vi "Upload File to Bucket.vi"() -> ()   [LabVIEW 2015]
doc: "Demonstrates how to upload a file from the local file system to an Amazon S3 bucket."
uses:
  <vilib>/AWS Toolkit/Core/HTTP Request/AWS Credentials.ctl
  <vilib>/AWS Toolkit/S3/ACL.ctl
  <vilib>/AWS Toolkit/S3/PUT Object Request Parameters.ctl
  <vilib>/AWS Toolkit/S3/Storage Class.ctl
  <vilib>/AWS Toolkit/Core/HTTP Request/Name Value Pair.ctl
  <vilib>/AWS Toolkit/Core/HTTP Request/HTTP Request.lvclass
  <vilib>/AWS Toolkit/S3/Bucket/Bucket.lvclass
  <vilib>/AWS Toolkit/S3/NI_AWS_S3.lvlib
panel:
  in  "File to Upload":path
  in  "Secret Key":string
  in  "Access Key":string
  out "New Object Location":string
  in  "Public":bool
  in  "Object Path":string="uploads/"
  in  "Destination Bucket":string
  # "Overview: Demonstrates how to upload a file to an Amazon S3 bucket.\nRequirements: NI Cloud Toolkit for AWS and a registered Amazon AWS account\nInstructions:\n1. Specify the Access Key and Secret Key for your AWS account. You can create an account at http://aws.amazon.com.\n2. Specify a Destination Bucket for the file. If you have not created a bucket, you can run the Create New Bucket.vi example to create a new bucket.\n3. Set Public to TRUE if you want the file to be public.\n4. Specify the File to Upload.\n5. Set the Object Path if you want to store the file in a folder within the bucket.\n6. Run the VI. Observe the URL of the stored file in the New Object Location indicator."
  # "Note: If you set Public to FALSE, you will not be able to download the file using the New Object Location URL. This is because you must use an authentication method to access non-public objects."
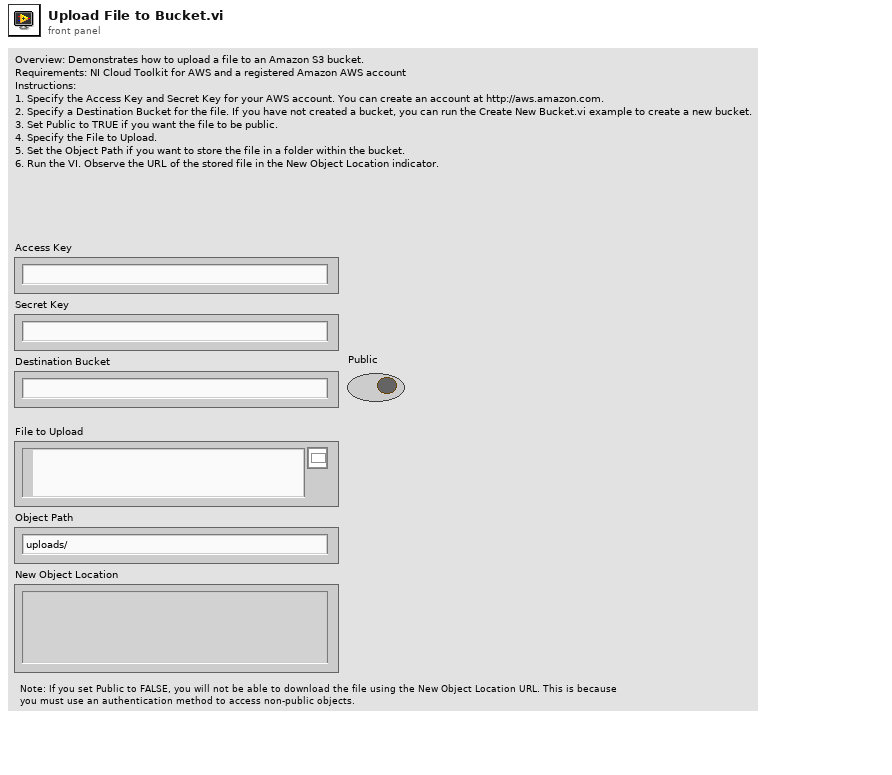
[diagram p1: front panel]
types:
  T1 = typedef "NI_AWS_Core.lvlib/HTTP Request.lvclass/AWS Credentials.ctl" = cluster{"Access Key":string, "Secret Key":string}
  T2 = typedef "NI_AWS_S3.lvlib/ACL.ctl" = enum16{"private", "public-read", "public-read-write", "aws-exec-read", "authenticated-read", "bucket-owner-read", "bucket-owner-full-control"}
  T3 = typedef "NI_AWS_S3.lvlib/PUT Object Request Parameters.ctl" = cluster{"Content Type":string, "ACL":T2, "Storage Class":T4, "User-Defined Metadata":T5[]}
  T4 = typedef "NI_AWS_S3.lvlib/Storage Class.ctl" = enum16{"STANDARD", "REDUCED_REDUNDANCY"}
  T5 = typedef "NI_AWS_Core.lvlib/HTTP Request.lvclass/Name Value Pair.ctl" = cluster{"name":string, "value":string}
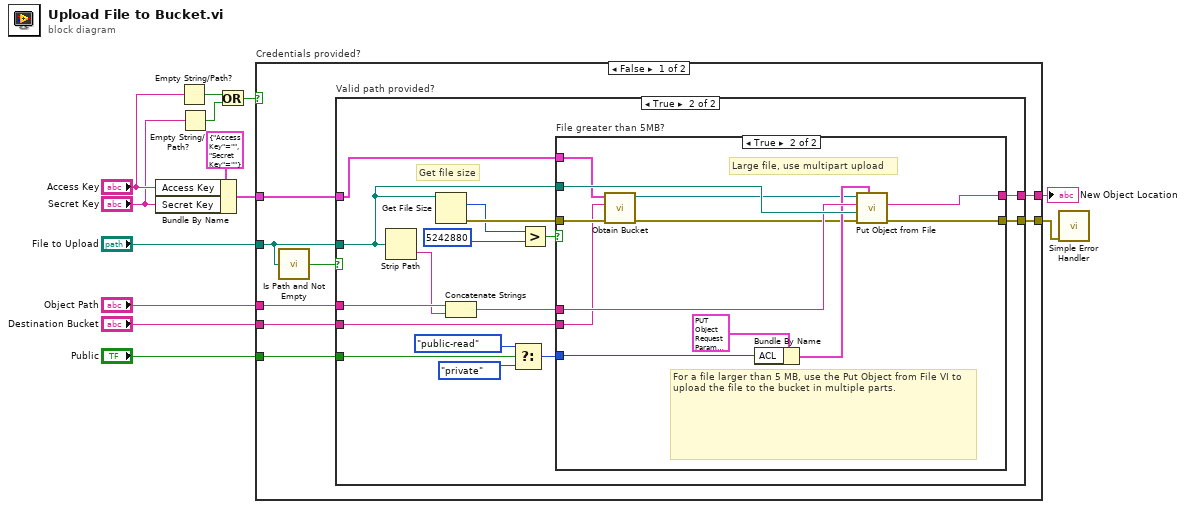
[diagram p0: block diagram]
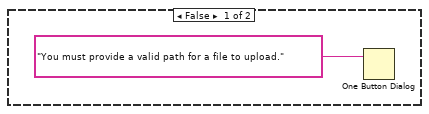
[diagram p2: hidden frame]
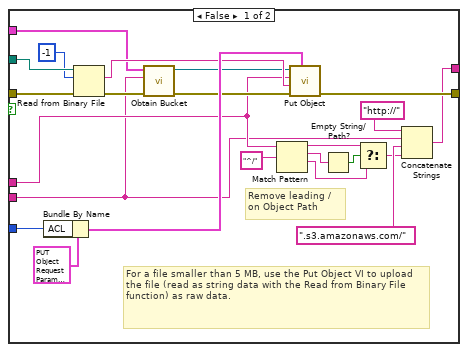
[diagram p3: hidden frame]
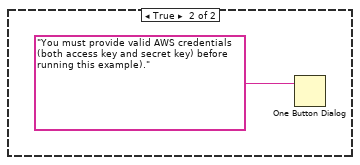
[diagram p4: hidden frame]
diagram:
  n1 = Bundle By Name(cluster=T1 {"Access Key"="", "Secret Key"=""} ("AWS Credentials in"), "Access Key"="Access Key", "Secret Key"="Secret Key") -> (w6:T1)
  n2 = Empty String/Path?(string/path="Access Key") -> (empty?=w11:bool)
  n3 = Empty String/Path?(string/path="Secret Key") -> (empty?=w12:bool)
  n4 = Or(x=w11, y=w12) -> (x .or. y?=w7:bool)
  n5 = case "Credentials provided?" shown="False" w7 {
    tunnel: w6 -> [w20 _]
    tunnel: [w21 _] -> w13
    tunnel: "File to Upload" -> [w19 _]
    tunnel: "Destination Bucket" -> [w17 _]
    tunnel: "Public" -> [w16 _]
    tunnel: "Object Path" -> [w15 _]
    tunnel: [w14 _] -> w1
    frame False {
      n6 = call <vilib>:"Is Path and Not Empty.vi"("path"=w19) -> ("Is Path and Not Empty?"=w18:bool)  [unwired: 4 in]
      n7 = case "Valid path provided?" shown="True" w18 {
        tunnel: w20 -> [_ w23]
        tunnel: w19 -> [_ w27]
        tunnel: [_ w38] -> w21
        tunnel: w17 -> [_ w32]
        tunnel: w16 -> [_ w31]
        tunnel: w15 -> [_ w30]
        tunnel: [_ w26] -> w14
        frame False {
          n8 = One Button Dialog(message="You must provide a valid path for a file to upload.") -> ()  [unwired: 1 in, 1 out]
        }
        frame True {
          # "Get file size"
          n9 = Strip Path(path=w27) -> (name=w28:string)  [unwired: 1 out]
          n10 = Get File Size(file=w27) -> (size (in bytes)=w36:i64, 0:w37:errorcluster)  [unwired: 1 in, 1 out]
          n11 = Concatenate Strings(w30, w28) -> (w29:string)
          n12 = Select(t=ACL."public-read" ("ACL"), s=w31, f=ACL."private" ("ACL")) -> (s? t:f=w33:T2)
          n13 = Greater?(x=w36, y=i64 5242880) -> (0:w34:bool)
          n14 = case "File greater than 5MB?" shown="True" w34 {
            tunnel: w37 -> [w61 w73]
            tunnel: w27 -> [w60 w72]
            tunnel: w32 -> [w40 w63]
            tunnel: w29 -> [w41 w71]
            tunnel: w33 -> [w58 w69]
            tunnel: [w56 w70] -> w26
            tunnel: [w53 w68] -> w38
            tunnel: w23 -> [w42 w64]
            frame False {
              # "Remove leading / \non Object Path"
              # "For a file smaller than 5 MB, use the Put Object VI to upload the file (read as string data with the Read from Binary File function) as raw data."
              n15 = Bundle By Name(cluster=T3 {"Content Type"="binary/octet-stream", "ACL"=enum."private", "Storage Class"=enum."STANDARD", "User-Defined Metadata"=[]} ("PUT Object Request Parameters"), "ACL"=w58) -> (w57:T3)
              n16 = Read from Binary File(8:w61, 10:-1 ("count (1)"), 11:w60) -> (0:w44:errorcluster, 2:w45:string)  [unwired: 3 in, 2 out]
              n17 = call <vilib>:"Obtain Bucket.vi"("error in (no error)"=w44, "Bucket name"=w40, "AWS Credentials"=w42) -> ("error out"=w43:errorcluster, "Bucket"=w39:refnum<class "Bucket.lvclass">)  [unwired: 7 in]
              n18 = Match Pattern(string=w41, regular expression="^/") -> (before substring=w51:string, match substring=w49:string, after substring=w52:string)  [unwired: 1 in, 1 out]
              n19 = call <vilib>:"Put Object.vi"("Object Parameters"=w57, "error in (no error)"=w43, "Object Data"=w45, "Object Path"=w41, "Bucket in"=w39) -> ("error out"=w56:errorcluster)  [unwired: 5 in, 1 out]
              n20 = Empty String/Path?(string/path=w49) -> (empty?=w50:bool)
              n21 = Select(t=w51, s=w50, f=w52) -> (s? t:f=w47:string)
              n22 = Concatenate Strings("http://" ("string"), w40, ".s3.amazonaws.com/" ("string"), w47) -> (w53:string)
            }
            frame True {
              # "For a file larger than 5 MB, use the Put Object from File VI to upload the file to the bucket in multiple parts."
              # "Large file, use multipart upload"
              n23 = call <vilib>:"Obtain Bucket.vi"("error in (no error)"=w73, "Bucket name"=w63, "AWS Credentials"=w64) -> ("error out"=w65:errorcluster, "Bucket"=w62:refnum<class "Bucket.lvclass">)  [unwired: 7 in]
              n24 = Bundle By Name(cluster=T3 {"Content Type"="binary/octet-stream", "ACL"=enum."private", "Storage Class"=enum."STANDARD", "User-Defined Metadata"=[]} ("PUT Object Request Parameters"), "ACL"=w69) -> (w66:T3)
              n25 = call <vilib>:"Put Object from File.vi"("Object Parameters"=w66, "error in (no error)"=w65, "File"=w72, "Object Path"=w71, "Bucket in"=w62) -> ("error out"=w70:errorcluster, "Location"=w68:string)  [unwired: 2 in, 3 out]
            }
          }
        }
      }
    }
    frame True {
      n26 = One Button Dialog(message="You must provide valid AWS credentials (both access key and secret key) before running this example).") -> ()  [unwired: 1 in, 1 out]
    }
  }
  "New Object Location" <- w13
  n27 = call <vilib>:"Simple Error Handler.vi"("error in (no error)"=w1) -> ()  [unwired: 4 in, 5 out]
